vi "ExtraFilter_4channel.vi"(5 "new coeffs":fxp<+/-,18,18>[](array[numeric]), 6 "reset":bool, 7 "new coeffs":bool, 8 "valid in":bool, 9 "enable filter":bool, 10 "new shift":i32, 11 "Data in":fxp<+/-,16,14>[](array[numeric])=[0.0, 0.0, 0.0, 0.0, 0.0, 0.0, 0.0, 0.0]) -> (0 "valid out":bool, 2 "Element2":u64, 3 "Element1":u64)   [LabVIEW 2013]
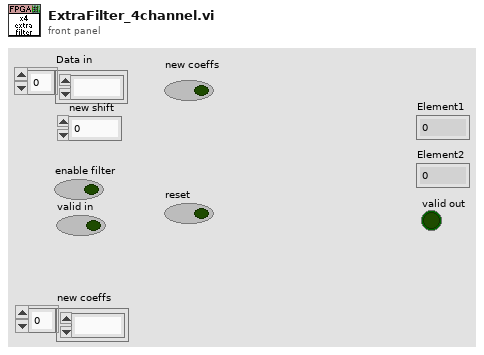
[diagram p1: front panel]
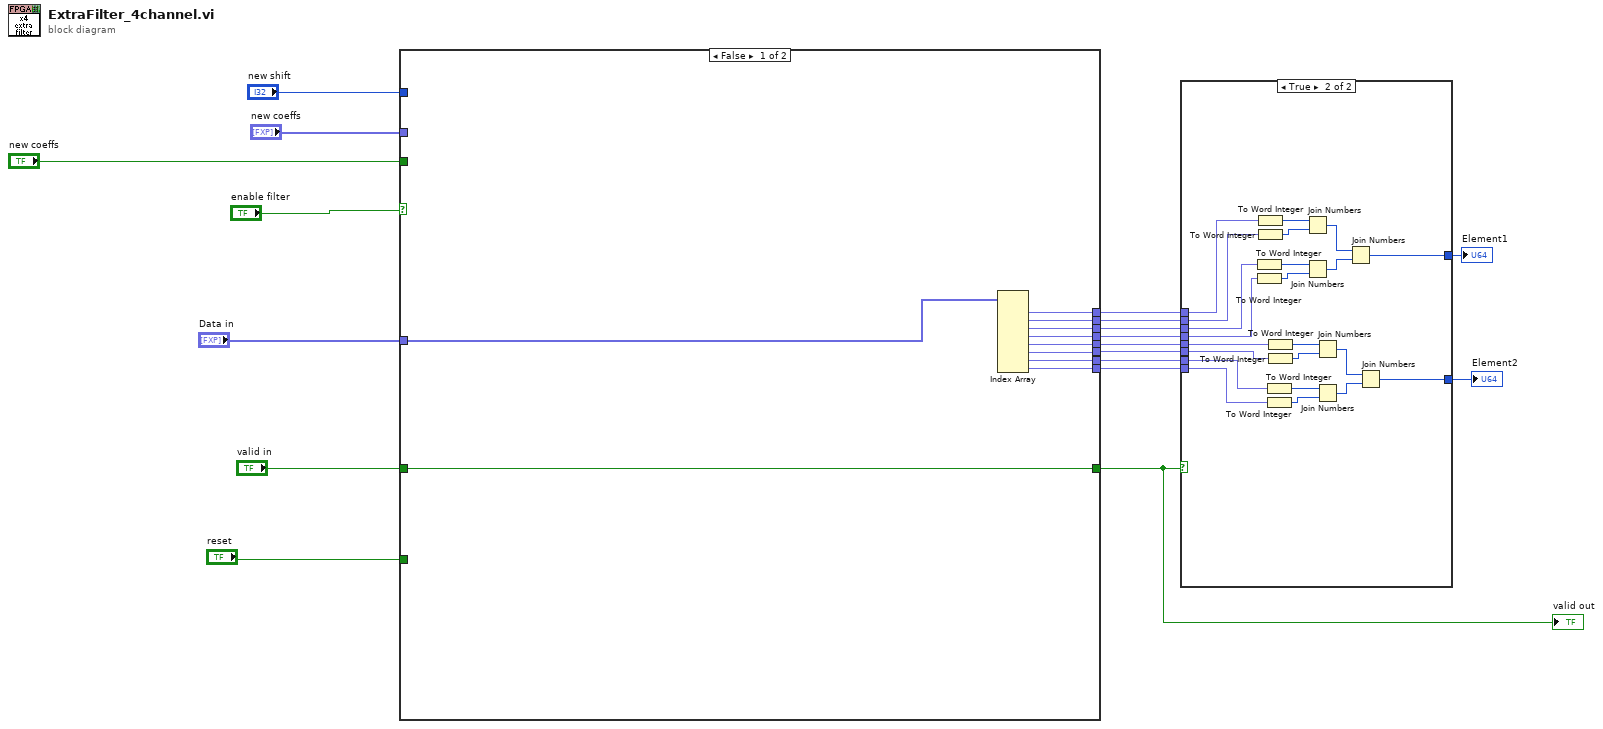
[diagram p0: block diagram]
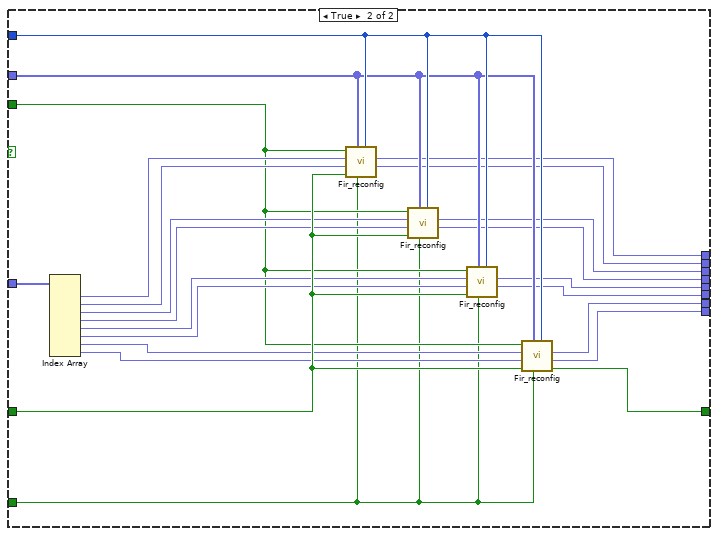
[diagram p3: hidden frame]
diagram:
  n1 = case shown="False" "enable filter" {
    tunnel: "Data in" -> [w26 w51]
    tunnel: "valid in" -> [w28 w50]
    tunnel: "new coeffs" -> [_ w38]
    tunnel: [w28 w49] -> w11
    tunnel: "new shift" -> [_ w39]
    tunnel: "new coeffs" -> [_ w40]
    tunnel: "reset" -> [_ w37]
    tunnel: [w27 w36] -> w10
    tunnel: [w25 w35] -> w9
    tunnel: [w24 w34] -> w8
    tunnel: [w23 w33] -> w7
    tunnel: [w21 w32] -> w6
    tunnel: [w22 w31] -> w5
    tunnel: [w20 w30] -> w4
    tunnel: [w19 w29] -> w3
    frame False {
      n2 = Index Array(array=w26) -> (element #1=w27:fxp<+/-,16,14>, element #2=w25:fxp<+/-,16,14>, element #3=w24:fxp<+/-,16,14>, element #4=w23:fxp<+/-,16,14>, element #5=w21:fxp<+/-,16,14>, element #6=w22:fxp<+/-,16,14>, element #7=w20:fxp<+/-,16,14>, element #8=w19:fxp<+/-,16,14>)  [unwired: 8 in]
    }
    frame True {
      n3 = Index Array(array=w51) -> (element #1=w48:fxp<+/-,16,14>, element #2=w47:fxp<+/-,16,14>, element #3=w46:fxp<+/-,16,14>, element #4=w45:fxp<+/-,16,14>, element #5=w44:fxp<+/-,16,14>, element #6=w43:fxp<+/-,16,14>, element #7=w42:fxp<+/-,16,14>, element #8=w41:fxp<+/-,16,14>)  [unwired: 8 in]
      n4 = call "Fir_reconfig.vi"("new shift"=w39, "reset"=w37, 7:"new coeffs"=w38, "valid in"=w50, "Q in"=w47, "I in"=w48, 11:"new coeffs"=w40) -> ("Q out"=w35:fxp<+/-,16,14>, "I out"=w36:fxp<+/-,16,14>)  [unwired: 1 in, 2 out]
      n5 = call "Fir_reconfig.vi"("new shift"=w39, "reset"=w37, 7:"new coeffs"=w38, "valid in"=w50, "Q in"=w45, "I in"=w46, 11:"new coeffs"=w40) -> ("Q out"=w33:fxp<+/-,16,14>, "I out"=w34:fxp<+/-,16,14>)  [unwired: 1 in, 2 out]
      n6 = call "Fir_reconfig.vi"("new shift"=w39, "reset"=w37, 7:"new coeffs"=w38, "valid in"=w50, "Q in"=w43, "I in"=w44, 11:"new coeffs"=w40) -> ("Q out"=w31:fxp<+/-,16,14>, "I out"=w32:fxp<+/-,16,14>)  [unwired: 1 in, 2 out]
      n7 = call "Fir_reconfig.vi"("new shift"=w39, "reset"=w37, 7:"new coeffs"=w38, "valid in"=w50, "Q in"=w41, "I in"=w42, 11:"new coeffs"=w40) -> ("valid out"=w49:bool, "Q out"=w29:fxp<+/-,16,14>, "I out"=w30:fxp<+/-,16,14>)  [unwired: 1 in, 1 out]
    }
  }
  "valid out" <- w11
  n8 = case shown="True" w11 {
    tunnel: w10 -> [_ w67]
    tunnel: w9 -> [_ w66]
    tunnel: w8 -> [_ w65]
    tunnel: w7 -> [_ w64]
    tunnel: w6 -> [_ w55]
    tunnel: w5 -> [_ w54]
    tunnel: w4 -> [_ w53]
    tunnel: w3 -> [_ w52]
    tunnel: [_ w63] -> w2
    tunnel: [_ w62] -> w1
    frame False {
    }
    frame True {
      n9 = To Word Integer(number=w65) -> (16bit integer=w71:i16)
      n10 = To Word Integer(number=w64) -> (16bit integer=w70:i16)
      n11 = To Word Integer(number=w67) -> (16bit integer=w72:i16)
      n12 = To Word Integer(number=w66) -> (16bit integer=w73:i16)
      n13 = To Word Integer(number=w53) -> (16bit integer=w58:i16)
      n14 = To Word Integer(number=w52) -> (16bit integer=w59:i16)
      n15 = To Word Integer(number=w55) -> (16bit integer=w57:i16)
      n16 = To Word Integer(number=w54) -> (16bit integer=w56:i16)
      n17 = Join Numbers(hi=w72, lo=w73) -> ((hi.lo)=w69:u32)
      n18 = Join Numbers(hi=w71, lo=w70) -> ((hi.lo)=w68:u32)
      n19 = Join Numbers(hi=w57, lo=w56) -> ((hi.lo)=w60:u32)
      n20 = Join Numbers(hi=w58, lo=w59) -> ((hi.lo)=w61:u32)
      n21 = Join Numbers(hi=w69, lo=w68) -> ((hi.lo)=w63:u64)
      n22 = Join Numbers(hi=w60, lo=w61) -> ((hi.lo)=w62:u64)
    }
  }
  "Element1" <- w2
  "Element2" <- w1
